vi "setServoArduinoNew.vi"(0 "speed":i32, 1 "Pulse Width in uS":u16=1500, 2 "servo id":i32) -> ()   [LabVIEW 2012]
uses:
  GlobalArduinoNew.vi
  <vilib>/LabVIEW Interface for Arduino/LabVIEW Interface for Arduino.lvlib
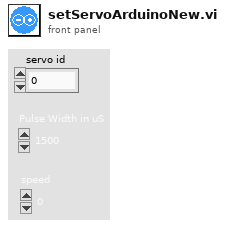
[diagram p1: front panel]
types:
  T1 = typedef "LabVIEW Interface for Arduino.lvlib/Arduino Resource.ctl" = cluster{"VISA resource":refnum<visa-resource-name>, "Board Type":T2, "Connection Type":enum8{"USB / Serial"}, "Bytes Per Packet (15)":u8}
  T2 = typedef "LabVIEW Interface for Arduino.lvlib/Board Type.ctl" = enum16{"Uno", "Dimuelanove w/Atmega 328", "Mega 2560"}
  T3 = typedef "Semaphore RefNum" = refnum<k1>
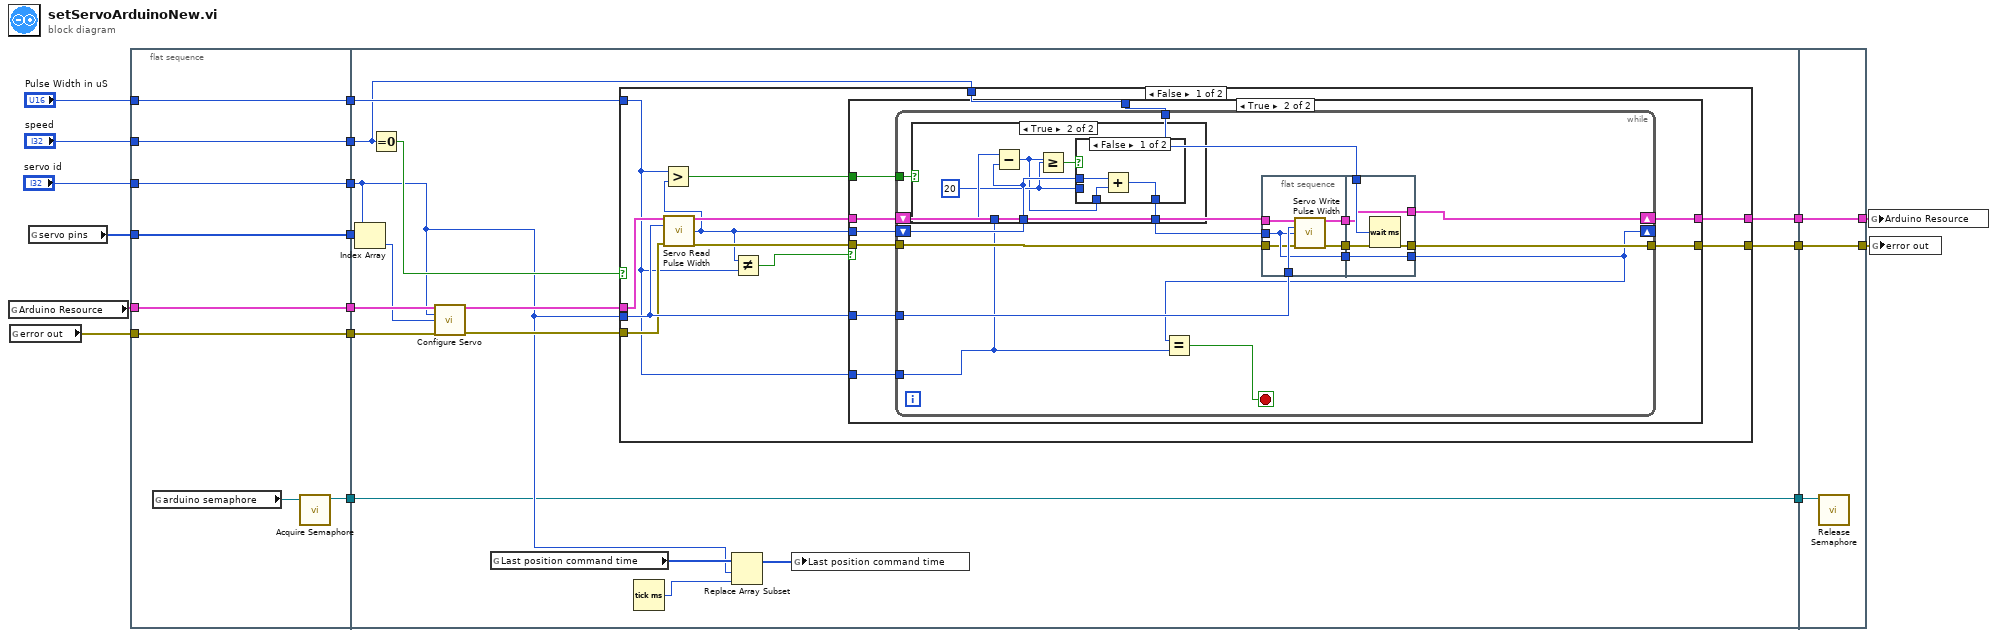
[diagram p0: block diagram]
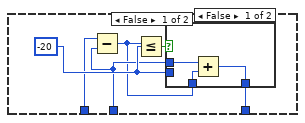
[diagram p3: hidden frame]
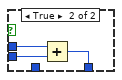
[diagram p4: hidden frame]
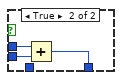
[diagram p5: hidden frame]
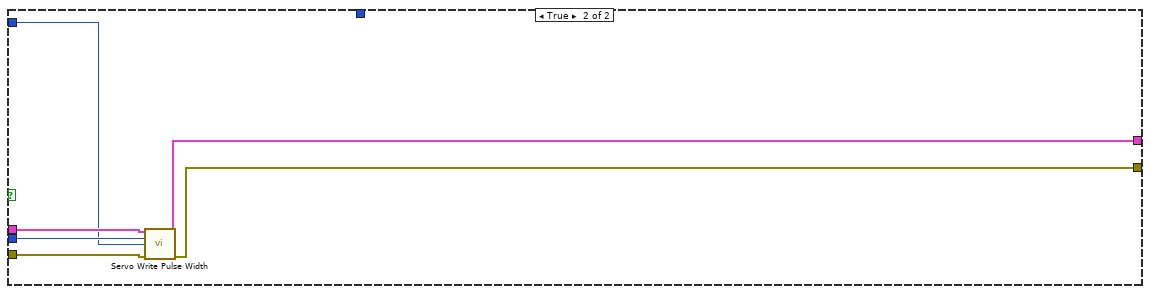
[diagram p6: hidden frame]
diagram:
  n1 = global read "GlobalArduinoNew.vi" "Arduino Resource"() -> (w18:T1)
  n2 = global read "GlobalArduinoNew.vi" "error out"() -> (w17:errorcluster)
  n3 = global read "GlobalArduinoNew.vi" "servo pins"() -> (w16:u8[])
  n4 = flat-sequence {
    tunnel: "servo id" -> [w21]
    tunnel: "speed" -> [w22]
    tunnel: "Pulse Width in uS" -> [w23]
    tunnel: w16 -> [w24]
    tunnel: w17 -> [w25]
    tunnel: w18 -> [w26]
    tunnel: [w26] -> w10
    tunnel: [w25] -> w9
    tunnel: [w24] -> w8
    tunnel: [w23] -> w7
    tunnel: [w22] -> w6
    tunnel: [w21] -> w5
    tunnel: [w19] -> w2
    tunnel: w10 -> [w41]
    tunnel: w9 -> [w40]
    tunnel: w8 -> [w37]
    tunnel: w7 -> [w35]
    tunnel: w6 -> [w34]
    tunnel: w5 -> [w29]
    tunnel: [w33] -> w4
    tunnel: [w32] -> w3
    tunnel: w2 -> [w27]
    tunnel: [w27] -> w1
    tunnel: [w122] -> w12
    tunnel: [w123] -> w13
    tunnel: w4 -> [w123]
    tunnel: w3 -> [w122]
    tunnel: w1 -> [w121]
    frame #0 {
      n5 = global read "GlobalArduinoNew.vi" "arduino semaphore"() -> (w20:T3)
      n6 = call <vilib>:"Acquire Semaphore.vi"("semaphore"=w20) -> ("semaphore out"=w19:T3)  [unwired: 4 in, 2 out]
    }
    frame #1 {
      n7 = Index Array(array=w37, index=w29) -> (element=w38:u8)
      n8 = Equal To 0?(x=w34) -> (x = 0?=w36:bool)
      n9 = call <vilib>:"Configure Servo.vi"("Arduino Resource"=w41, "Servo Number (0)"=w29, "DIO Pin (2)"=w38, "error in"=w40) -> ("Arduino Resource"=w42:T1, "error out"=w39:errorcluster)  [unwired: 10 in]
      n10 = global read "GlobalArduinoNew.vi" "Last position command time"() -> (w30:u64[])
      n11 = case shown="False" w36 {
        tunnel: w42 -> [w53 w120]
        tunnel: w39 -> [w46 w119]
        tunnel: w29 -> [w50 w118]
        tunnel: w35 -> [w43 w117]
        tunnel: w34 -> [w51 _]
        tunnel: [w49 w115] -> w33
        tunnel: [w48 w116] -> w32
        frame False {
          n12 = call <vilib>:"Servo Read Pulse Width.vi"("Arduino Resource"=w53, "Servo Number"=w50, "error in"=w46) -> ("Arduino Resource"=w54:T1, "Pulse Width in uS"=w44:u16, "error out"=w47:errorcluster)  [unwired: 10 in]
          n13 = Greater?(x=w43, y=w44) -> (0:w52:bool)
          n14 = Not Equal?(x=w44, y=w43) -> (x != y?=w45:bool)
          n15 = case shown="True" w45 {
            tunnel: w54 -> [w56 w65]
            tunnel: w43 -> [_ w64]
            tunnel: w44 -> [_ w63]
            tunnel: w52 -> [_ w62]
            tunnel: w51 -> [_ w61]
            tunnel: w50 -> [_ w60]
            tunnel: [w56 w59] -> w49
            tunnel: [w55 w58] -> w48
            tunnel: w47 -> [w55 w57]
            frame False {
            }
            frame True {
              n16 = while {
                tunnel: w64 -> [w66]
                shift-right: [w72] -> w59
                shift-left: w65 -> [w76]
                shift-right: [w67] -> _
                shift-left: w63 -> [w78]
                tunnel: w62 -> [w79]
                tunnel: w61 -> [w77]
                tunnel: w60 -> [w74]
                tunnel: [w69] -> w58
                tunnel: w57 -> [w68]
                stop <- w80 stop-if-true
                n17 = case shown="True" w79 {
                  tunnel: w78 -> [w93 w106]
                  tunnel: [w92 w105] -> w75
                  tunnel: w66 -> [w94 w108]
                  frame False {
                    w95 = i16 -20 ("y")
                    n18 = Subtract(x=w94, y=w93) -> (x-y=w91:u16)
                    n19 = Less Or Equal?(x=w91, y=w95) -> (x <= y?=w96:bool)
                    n20 = case shown="False" w96 {
                      tunnel: w93 -> [w99 w102]
                      tunnel: w95 -> [_ w101]
                      tunnel: [w98 w100] -> w92
                      tunnel: w91 -> [w97 _]
                      frame False {
                        n21 = Add(x=w99, y=w97) -> (x+y=w98:u16)
                      }
                      frame True {
                        n22 = Add(x=w102, y=w101) -> (x+y=w100:u16)
                      }
                    }
                  }
                  frame True {
                    w104 = u16 20 ("y")
                    n23 = Subtract(x=w108, y=w106) -> (x-y=w103:u16)
                    n24 = Greater Or Equal?(x=w103, y=w104) -> (x >= y?=w107:bool)
                    n25 = case shown="False" w107 {
                      tunnel: w106 -> [w111 w114]
                      tunnel: w104 -> [_ w113]
                      tunnel: [w110 w112] -> w105
                      tunnel: w103 -> [w109 _]
                      frame False {
                        n26 = Add(x=w111, y=w109) -> (x+y=w110:u16)
                      }
                      frame True {
                        n27 = Add(x=w114, y=w113) -> (x+y=w112:u16)
                      }
                    }
                  }
                }
                n28 = Equal?(x=w67, y=w66) -> (x = y?=w80:bool)
                n29 = flat-sequence {
                  tunnel: w76 -> [w86]
                  tunnel: w75 -> [w83]
                  tunnel: w74 -> [w85]
                  tunnel: [w84] -> w73
                  tunnel: [w83] -> w71
                  tunnel: [w82] -> w70
                  tunnel: w68 -> [w81]
                  tunnel: w77 -> [w90]
                  tunnel: w73 -> [w89]
                  tunnel: [w89] -> w72
                  tunnel: [w88] -> w67
                  tunnel: w71 -> [w88]
                  tunnel: w70 -> [w87]
                  tunnel: [w87] -> w69
                  frame #0 {
                    n30 = call <vilib>:"Servo Write Pulse Width.vi"("Arduino Resource"=w86, "Servo Number"=w85, "Pulse Width in uS"=w83, "error in"=w81) -> ("Arduino Resource"=w84:T1, "error out"=w82:errorcluster)  [unwired: 10 in]
                  }
                  frame #1 {
                    n31 = Wait (ms)(milliseconds to wait=w90) -> ()  [unwired: 1 out]
                  }
                }
              }
            }
          }
        }
        frame True {
          n32 = call <vilib>:"Servo Write Pulse Width.vi"("Arduino Resource"=w120, "Servo Number"=w118, "Pulse Width in uS"=w117, "error in"=w119) -> ("Arduino Resource"=w115:T1, "error out"=w116:errorcluster)  [unwired: 10 in]
        }
      }
      n33 = Tick Count (ms)() -> (millisecond timer value=w28:u32)
      n34 = Replace Array Subset(array=w30, new element=w28, index=w29) -> (w31:u64[])
      n35 = global write "GlobalArduinoNew.vi" "Last position command time"(w31) -> ()
    }
    frame #2 {
      n36 = call <vilib>:"Release Semaphore.vi"("semaphore"=w121) -> ()  [unwired: 5 in, 2 out]
    }
  }
  n37 = global write "GlobalArduinoNew.vi" "Arduino Resource"(w13) -> ()
  n38 = global write "GlobalArduinoNew.vi" "error out"(w12) -> ()
